vi "FTW-NUM-Counter.vi"(1 "Reset?":bool) -> (0 "Counter":i32 format="%08x")   [LabVIEW 2014]
panel:
  # "Inputs"
  # "Outputs"
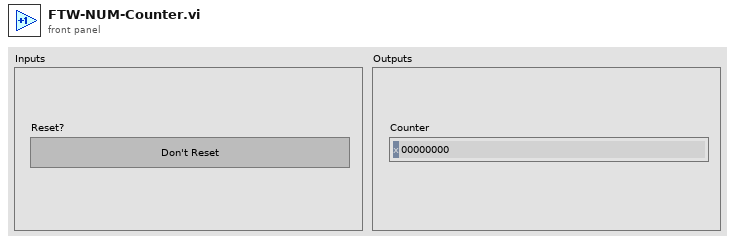
[diagram p1: front panel]
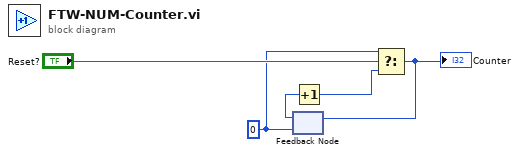
[diagram p0: block diagram]
diagram:
  w3 = 0
  n1 = feedback #1(w3) -> (w5:i32)
  n2 = Increment(x=w5) -> (x+1=w2:i32)
  n3 = Select(t=w3, s="Reset?", f=w2) -> (s? t:f=w1:i32)
  "Counter" <- w1
  n4 = feedback-in #1(w1) -> ()
